vi "Import Routing and Faulting Custom Device.vi"(8 "error in":errorcluster, 10 "datalog path (use dialog)":path, 11 "routing and faulting custom device in":T1 format="%.0x") -> (0 "error out":errorcluster, 3 "routing and faulting custom device out":T1 format="%.0x")   [LabVIEW 2020, in "Routing and Faulting Scripting.lvlib"]
doc: "Replaces the existing Routing and Faulting custom device configuration with the configuration specified by a datalog file. Create the datalog file by using <b>Export Routing and Faulting Custom Device.vi</b>."
uses:
  Routing and Faulting Scripting.lvlib
  <vilib>/NI/NI VeriStand Custom Device Import and Export Tool/ImportExport.lvlib
  <vilib>/NI VeriStand/Custom Device API/Custom Device Item Ref.ctl
  <vilib>/NI VeriStand/Custom Device API/Custom Device API.lvlib
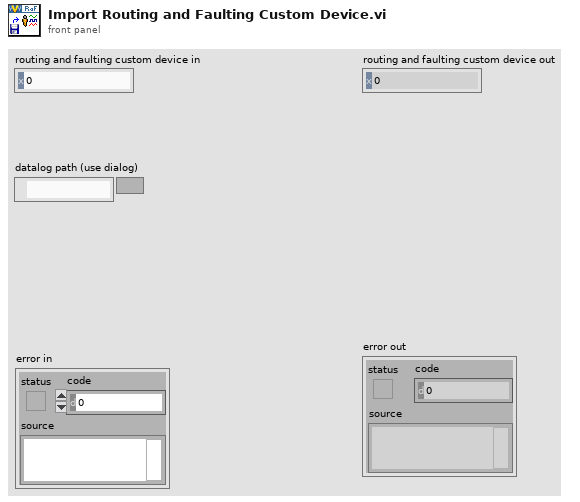
[diagram p1: front panel]
types:
  T1 = typedef "Custom Device API.lvlib/Custom Device Item Ref.ctl" = u64
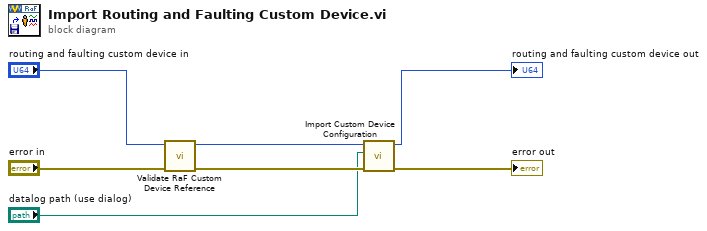
[diagram p0: block diagram]
diagram:
  n1 = call "Validate RaF Custom Device Reference.vi"("error in"="error in", "routing and faulting in"="routing and faulting custom device in") -> ("error out"=w4:errorcluster, "routing and faulting out"=w5:T1)  [unwired: 8 in]
  n2 = call <vilib>:"Import Custom Device Configuration.vi"("error in (no error)"=w4, "Path"="datalog path (use dialog)", "NodeID"=w5) -> ("error out"=→"error out":errorcluster, "NodeID out"=→"routing and faulting custom device out":u64)  [unwired: 6 in, 1 out]
